vi "Omni-Bus Inject U64.vi"(6 "Enable":bool, 8 "error in (no error)":errorcluster, 9 "Injected Value":u64, 10 "Tag":string, 11 "Omni_Bus in":refnum<class "Omni_Bus.lvclass">) -> (0 "error out":errorcluster, 3 "Omni_Bus out":refnum<class "Omni_Bus.lvclass">)   [LabVIEW 2021, in "Fault-Injection Bus.lvclass"]
uses:
  Fault-Injection Bus.lvclass
  Omni-Bus/Omni_Bus.lvclass
  Fault-Injection Bus.lvclass/Fault-Injection Bus.ctl
  Value Type/U64/Fault-Injection_U64.lvclass
  C:/Program Files (x86)/National Instruments/LabVIEW 2021/vi.lib/TSA/Abstract Data Classes/Abs_Types/Type/Abs_Type.lvclass
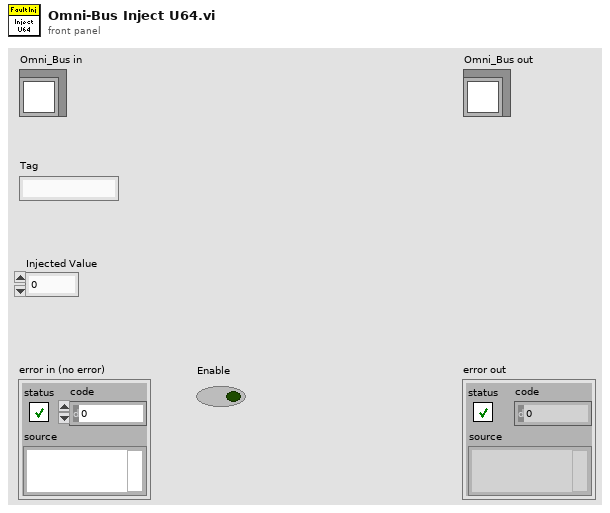
[diagram p1: front panel]
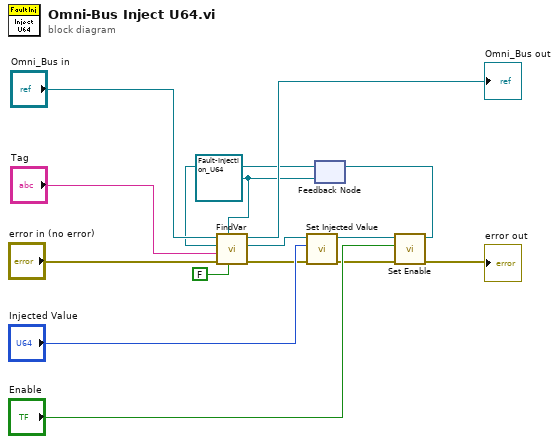
[diagram p0: block diagram]
diagram:
  w1 = refnum<class "Fault-Injection_U64.lvclass"> refnum ("Fault-Injection_Boolean out")
  n1 = feedback #1(w1) -> (w6:refnum<class "Fault-Injection_U64.lvclass">)
  n2 = call "FindVar.vi"("Write?"=FALSE, "Abs_Type"=w1, "error in (no error)"="error in (no error)", "Tag"="Tag", "Abs_Type Default"=w6, "Var Bus in"="Omni_Bus in") -> ("error out"=w8:errorcluster, "Abs_Type Found"=w7:refnum<class "Fault-Injection_U64.lvclass">, "Var Bus out"=→"Omni_Bus out":refnum<class "Omni_Bus.lvclass">)  [unwired: 2 in, 1 out]
  n3 = call-dynamic "Set Injected Value.vi"("error in (no error)"=w8, "Value"="Injected Value", "Fault-Injection_Boolean in"=w7) -> ("error out"=w5:errorcluster, "Fault-Injection_Boolean out"=w4:refnum<class "Fault-Injection_U64.lvclass">)  [unwired: 7 in]
  n4 = call-dynamic "Set Enable.vi"("error in (no error)"=w5, "Enable"="Enable", "Fault-Injection_Boolean in"=w4) -> ("error out"=→"error out":errorcluster, "Fault-Injection_Boolean out"=w3:refnum<class "Fault-Injection_U64.lvclass">)  [unwired: 7 in]
  n5 = feedback-in #1(w3) -> ()
